vi "AWS_ReadDataPlugins.vi"(8 "Error In":errorcluster, 11 "File Path Control":path) -> (0 "Error Out":errorcluster, 3 "Data Graph":dynamicdata(graph))   [LabVIEW 2014]
uses:
  <vilib>/Platform/storage/lvStorage.llb/_openFunction.ctl
  <vilib>/Platform/storage/lvStorage.llb/_openStorageWithRootAutoDetect.vi
  <vilib>/Platform/storage/lvStorage.llb/xStorage/xStorageSupp/ErrorOut.vi
  <vilib>/Platform/storage/lvStorage.llb/_queryPropPoly.vi
  <vilib>/Platform/storage/lvStorage.llb/_queryPropString.vi
  <vilib>/Platform/storage/lvStorage.llb/_queryGenericObjects.vi
  <vilib>/Platform/storage/lvStorage.llb/_loadAllDdt.vi
  <vilib>/Platform/storage/Storage.llb/Get Object Info.vi
  <vilib>/Platform/storage/Storage.llb/__closeStorageFromObject.vi
  <vilib>/Platform/storage/lvStorage.llb/xStorage/Open Data Storage/Open Data Storage.xnode
  <vilib>/Platform/storage/lvStorage.llb/xStorage/Read Data/Read Data.xnode
  <vilib>/Platform/storage/lvStorage.llb/xStorage/Close Data Storage/Close Data Storage.xnode
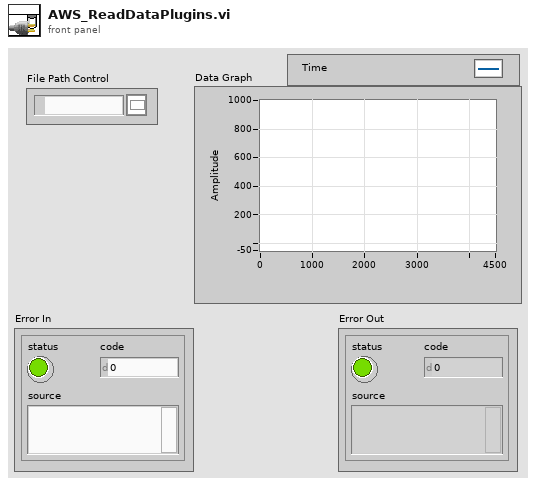
[diagram p1: front panel]
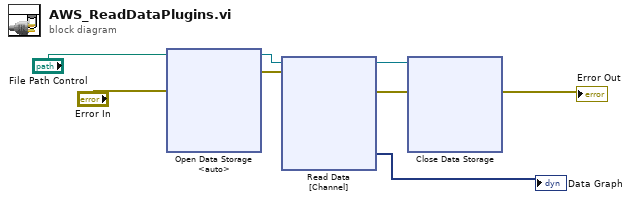
[diagram p0: block diagram]
diagram:
  n1 = xnode "Open Data Storage\n<auto>"("file path"="File Path Control", "error in (no error)"="Error In") -> ("storage refnum (file)"=w8:refnum<k20>, "error out"=w7:errorcluster)  [unwired: 3 in, 1 out]
  n2 = xnode "Read Data\n[Channel]"("storage refnum (file)"=w8, "error in"=w7) -> ("Signal"=→"Data Graph":dynamicdata, "storage refnum (file) out"=w6:refnum<k20>, "error out"=w5:errorcluster)  [unwired: 2 in, 1 out]
  n3 = xnode "Close Data Storage\n"("storage refnum (file)"=w6, "error in (no error)"=w5) -> ("error out"=→"Error Out":errorcluster)  [unwired: 1 out]
